vi "gps_speed_formula.vi"(6 "Latitude 2":dbl, 7 "Longitude 2":dbl, 9 "Time Delta":dbl, 10 "Longitude":dbl, 11 "Latitude":dbl) -> (3 "Speed":dbl)   [LabVIEW 2023]
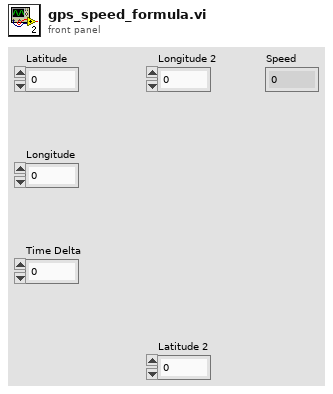
[diagram p1: front panel]
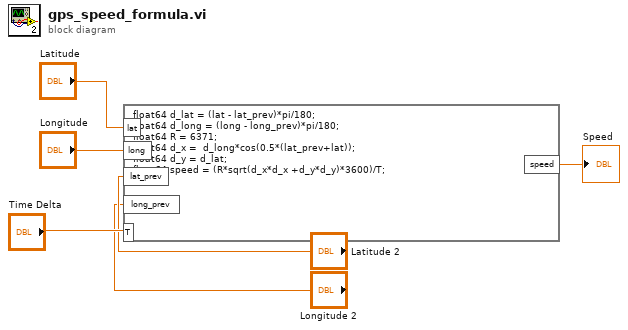
[diagram p0: block diagram]
diagram:
  n1 = formula code="float64 d_lat = (lat - lat_prev)*pi/180;\nfloat64 d_long = (long - long_prev)*pi/180;\nfloat64 R = 6371;\nfloat64 d_x =  d_long*cos(0.5*(lat_prev+lat));\nfloat64 d_y = d_lat;\nfloat64 speed = (R*sqrt(d_x*d_x +d_y*d_y)*3600)/T;"("lat"="Latitude", "lat_prev"="Latitude 2", "long"="Longitude", "long_prev"="Longitude 2", "T"="Time Delta") -> ("speed"=→"Speed":dbl)
